vi "Set Temperature (Celsius).vi"(8 "Error In":errorcluster, 10 "Temperature (Celsius)":dbl, 11 "Dual Mode Thermometer in":refnum<class "Dual Mode Thermometer.lvclass">) -> (0 "Error Out":errorcluster, 3 "Dual Mode Thermometer out":refnum<class "Dual Mode Thermometer.lvclass">)   [LabVIEW 2013, in "Dual Mode Thermometer.lvclass"]
doc: "Copyright (c) 2016 Sze Howe Koh\nThis code is licensed under the MIT license"
uses:
  Dual Mode Thermometer.lvclass
  Dual Mode Thermometer.lvclass/Dual Mode Thermometer.ctl
  src/LabVIEW/Qwt/QwtAbstractSlider/QwtAbstractSlider.lvclass
  src/LabVIEW/Qwt/QwtThermo/QwtThermo.lvclass
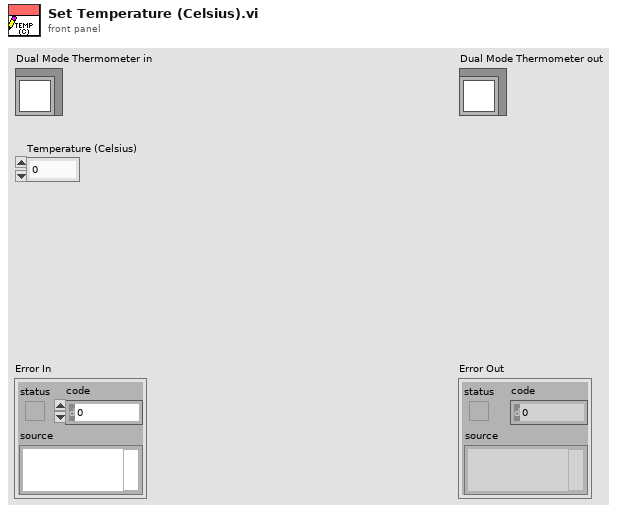
[diagram p1: front panel]
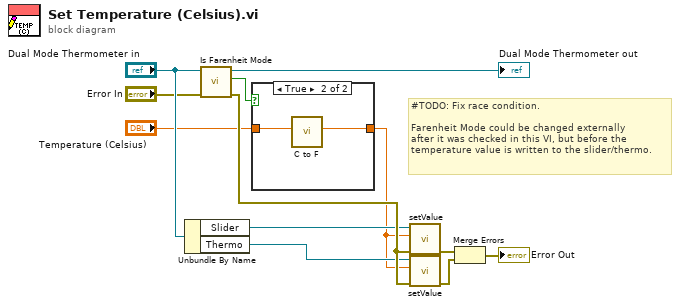
[diagram p0: block diagram]
diagram:
  # "#TODO: Fix race condition.\n\nFarenheit Mode could be changed externally\nafter it was checked in this VI, but before the \ntemperature value is written to the slider/thermo."
  n1 = Unbundle By Name("Dual Mode Thermometer in") -> ("Slider"=w9:refnum<class "QwtSlider.lvclass">, "Thermo"=w8:refnum<class "QwtThermo.lvclass">)
  n2 = call "Is Farenheit Mode.vi"("Error In"="Error In", "Dual Mode Thermometer In"="Dual Mode Thermometer in") -> ("Error Out"=w12:errorcluster, "Farenheit Mode"=w7:bool, "Dual Mode Thermometer out"=→"Dual Mode Thermometer out":refnum<class "Dual Mode Thermometer.lvclass">)  [unwired: 7 in]
  n3 = case shown="True" w7 {
    tunnel: "Temperature (Celsius)" -> [w13 w15]
    tunnel: [w13 w14] -> w5
    frame False {
    }
    frame True {
      n4 = call "C to F.vi"("Value [°C]"=w15) -> ("Value [°F]"=w14:dbl)  [unwired: 10 in]
    }
  }
  n5 = call "setValue.vi"("Error In"=w12, "val"=w5, "QwtAbstractSlider In"=w9) -> ("Error Out"=w3:errorcluster)  [unwired: 7 in, 1 out]
  n6 = call "setValue.vi"("Error In"=w12, "value"=w5, "QwtThermo In"=w8) -> ("Error Out"=w2:errorcluster)  [unwired: 7 in, 1 out]
  n7 = Merge Errors(w3, w2) -> (→"Error Out":errorcluster)
